vi "To String.vi"(7 "Pretty Print?":bool, 8 "error in (no error)":errorcluster, 11 "JSON Object in":refnum<class "JSON Object.lvclass">) -> (0 "error out":errorcluster, 3 "String":string)   [LabVIEW 2017, in "LVJSON.lvlib" / "JSON Object.lvclass"]
uses:
  JSON Object.lvclass
  JSON Object.lvclass/JSON Object.ctl
  JSON Datatype/JSON Datatype.lvclass
  LVJSON.lvlib
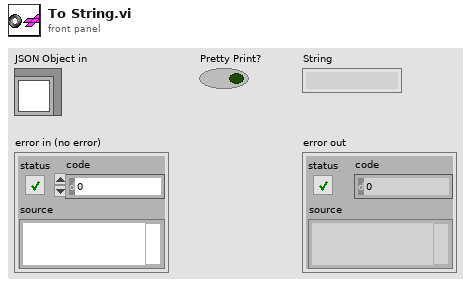
[diagram p1: front panel]
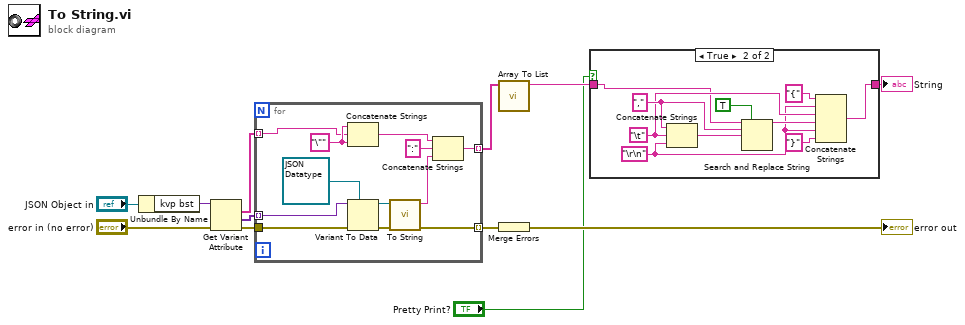
[diagram p0: block diagram]
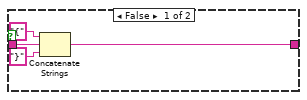
[diagram p2: hidden frame]
diagram:
  n1 = Unbundle By Name("JSON Object in") -> ("kvp bst"=w11:variant)
  n2 = Get Variant Attribute(Variant=w11, error in="error in (no error)") -> (names=w10:string[], values=w9:variant[], error out=w4:errorcluster)  [unwired: 2 in, 1 out]
  n3 = for {
    tunnel: w10 -> [w20] mode=indexing
    tunnel: w9 -> [w24] mode=indexing
    tunnel: [w22] -> w7 mode=indexing
    tunnel: w4 -> [w15]
    tunnel: [w13] -> w3 mode=indexing
    w21 = "\"" ("string")
    n4 = Concatenate Strings(w21, w20, w21) -> (w19:string)
    n5 = Variant To Data(error in=w15, type=refnum<class "JSON Datatype.lvclass"> refnum ("JSON Datatype.lvclass"), Variant=w24) -> (data=w17:refnum<class "JSON Datatype.lvclass">, error out=w14:errorcluster)
    n6 = call-dynamic "To String.vi"("error in (no error)"=w14, "JSON Datatype in"=w17) -> ("error out"=w13:errorcluster, "String"=w16:string)  [unwired: 8 in]
    n7 = Concatenate Strings(w19, ":" ("string"), w16) -> (w22:string)
  }
  n8 = call "Array To List.vi"("Array"=w7) -> ("String"=w6:string)  [unwired: 10 in]
  n9 = Merge Errors(w3) -> (→"error out":errorcluster)
  n10 = case shown="True" "Pretty Print?" {
    tunnel: [w26 w29] -> w8
    tunnel: w6 -> [w25 w30]
    frame False {
      n11 = Concatenate Strings("{" ("string"), w25, "}" ("string")) -> (w26:string)
    }
    frame True {
      w31 = "\r\n"
      w35 = "\t"
      w38 = "," ("search string")
      n12 = Concatenate Strings(w38, w35, w31) -> (w37:string)
      n13 = Search and Replace String(replace all?=TRUE ("replace all? (F)"), input string=w30, search string=w38, replace string=w37) -> (result string=w34:string)  [unwired: 4 in, 3 out]
      n14 = Concatenate Strings("{" ("string"), w31, w35, w34, w31, "}" ("string")) -> (w29:string)
    }
  }
  "String" <- w8
